vi "write_params.vi"(8 "error in (no error)":errorcluster, 10 "params":T1={"n_clusters"={"n_clusters_type"="euclidean", "n_clusters_int"=2.0}, "affinity"={"affinity_type"="euclidean", "affinity_function"="metric_function"}, "memory"="", "connectivity"={"connectivity_type"="None", "connectivity_list"=[]}, "compute_full_tree"={"compute_full_tree_type"="auto", "compute_full_tree_bool"=FALSE}, "linkage"="ward", "distance_threshold"={"distance_threshold_type"="None", "distance_threshold_float"=0.0}, "compute_distances"=FALSE}, 11 "AgglomerativeClustering in":refnum<class "AgglomerativeClustering.lvclass">) -> (0 "error out":errorcluster, 3 "AgglomerativeClustering out":refnum<class "AgglomerativeClustering.lvclass">)   [LabVIEW 2020, in "AgglomerativeClustering.lvclass"]
uses:
  AgglomerativeClustering.lvclass
  controls/agglomerative_clustering_params.ctl
  AgglomerativeClustering.lvclass/AgglomerativeClustering.ctl
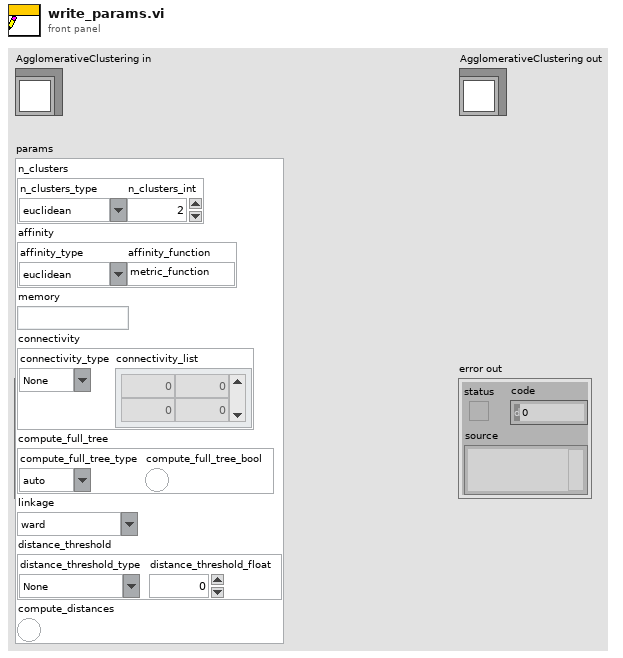
[diagram p1: front panel]
types:
  T1 = typedef "agglomerative_clustering_params.ctl" = cluster{"n_clusters":cluster{"n_clusters_type":string, "n_clusters_int":dbl}, "affinity":cluster{"affinity_type":string, "affinity_function":string}, "memory":string, "connectivity":cluster{"connectivity_type":string, "connectivity_list":dbl[][]}, "compute_full_tree":cluster{"compute_full_tree_type":string, "compute_full_tree_bool":bool}, "linkage":string, "distance_threshold":cluster{"distance_threshold_type":string, "distance_threshold_float":dbl}, "compute_distances":bool}
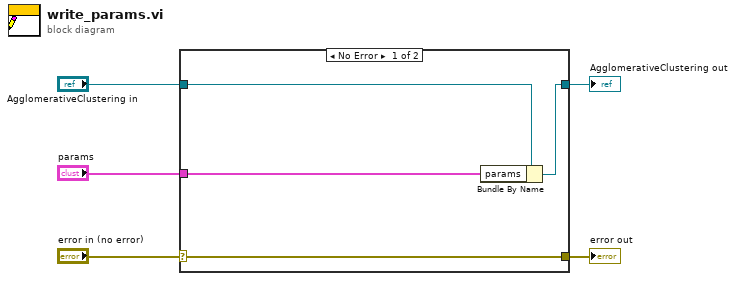
[diagram p0: block diagram]
diagram:
  n1 = case shown="No Error" "error in (no error)" {
    selector: "error in (no error)" -> [w9 w10]
    tunnel: [w9 w10] -> w4
    tunnel: [w7 w11] -> w2
    tunnel: "AgglomerativeClustering in" -> [w8 w11]
    tunnel: "params" -> [w6 _]
    frame No Error {
      n2 = Bundle By Name(cluster=w8, "params"=w6) -> (w7:refnum<class "AgglomerativeClustering.lvclass">)
    }
    frame Error {
    }
  }
  "error out" <- w4
  "AgglomerativeClustering out" <- w2
